vi "Untitled 3.vi"() -> ()   [LabVIEW 2014]
uses:
  Icons/Control 3.ctl
  Users/Yoerimartinez/Downloads/Control 5.ctl
  Icons/Control 6.ctl
  Icons/Control 7.ctl
panel:
  in  "Tab Control 3":enum32{"Page 1", "Page 2"}(tab)
  in  "Tab Control 2":enum32{"Page 1", "Page 2"}(tab)
  in  "Tab Control":T1
  in  "OK Button 3":T2
  out "Boolean":bool
  in  "OK Button 2":T3
  in  "Blank Button":T4
  in  "Numeric":dbl
  in  "OK Button":bool
  # "erwetwet"
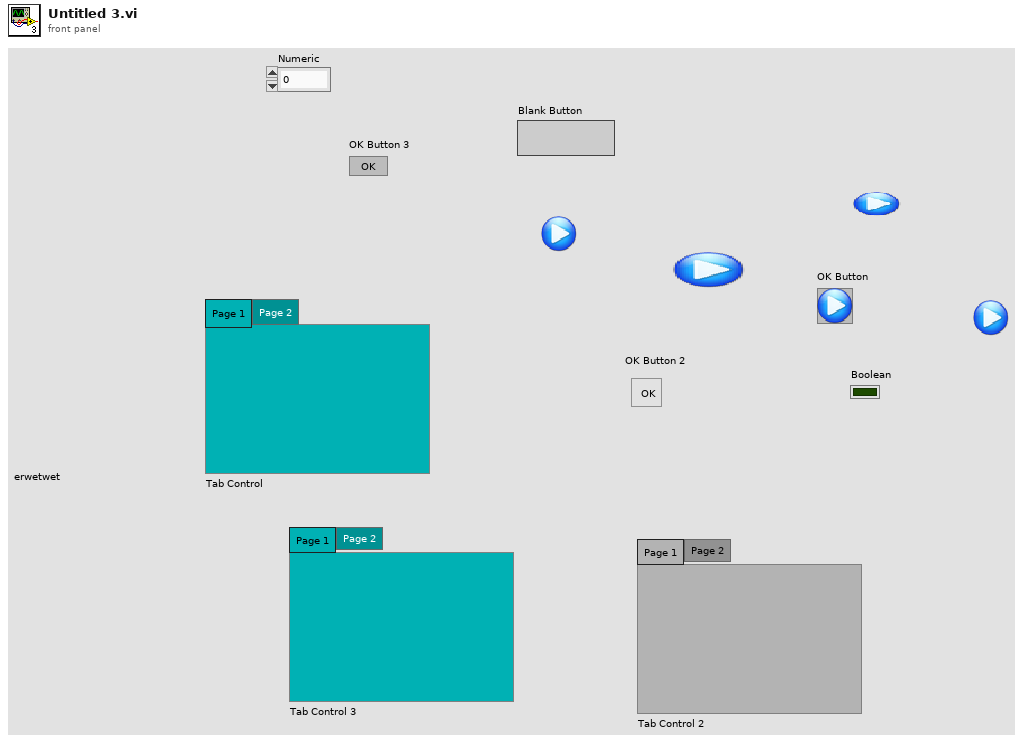
[diagram p1: front panel]
types:
  T1 = typedef "Control 7.ctl" = enum32{"Page 1", "Page 2"}
  T2 = typedef "Control 6.ctl" = bool
  T3 = typedef "Control 5.ctl" = bool
  T4 = typedef "Control 3.ctl" = bool
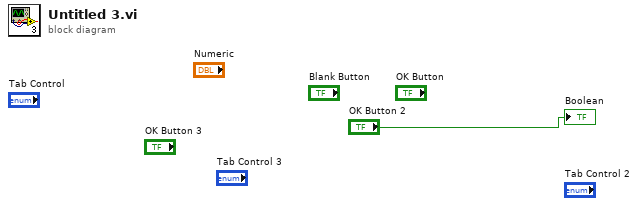
[diagram p0: block diagram]
diagram:
  "Boolean" <- "OK Button 2"
